vi "PH_Beckhoff_Application.declare digital PILS external InputTags.vi"() -> (0 "Digital Inputs":T2, 1 "Description":string)   [LabVIEW 2014, in "PH_Beckhoff_Application.lvlib"]
uses:
  PH_Beckhoff_Application.lvlib
  PH_Beckhoff/PH_Beckhoff.Digital Inputs.ctl
  PH_Beckhoff/PH_Beckhoff.lvlib
panel:
  in  "Digital Input Value":T1
  out "Right Size?":bool
  # "Let this VI run to check the size!"
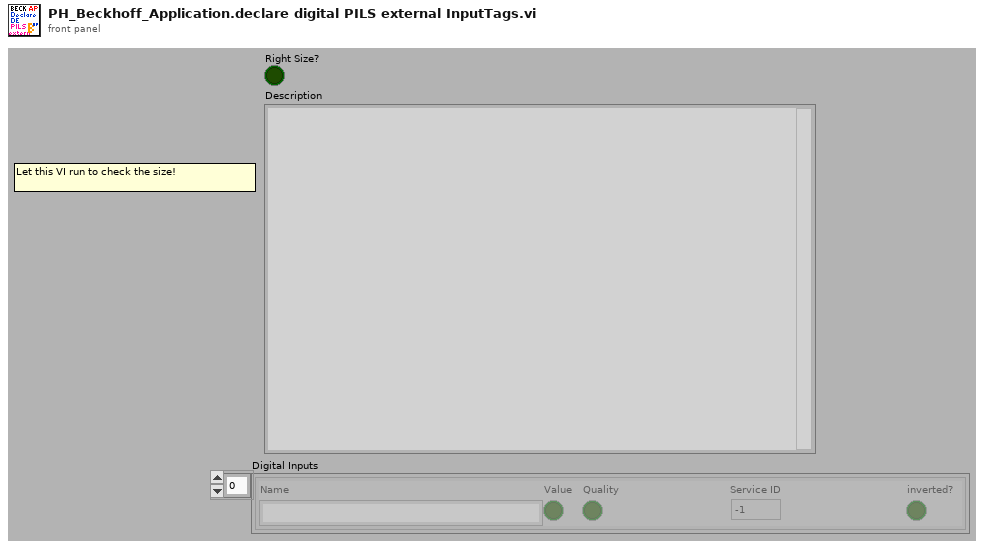
[diagram p1: front panel]
types:
  T1 = cluster{"Name":string, "Value":bool, "Quality":bool, "Service ID":i32, "inverted?":bool}
  T2 = typedef "PH_Beckhoff.lvlib/PH_Beckhoff.Digital Inputs.ctl" = cluster{"Name":string, "Value":bool, "Quality":bool, "Service ID":i32, "inverted?":bool}[]
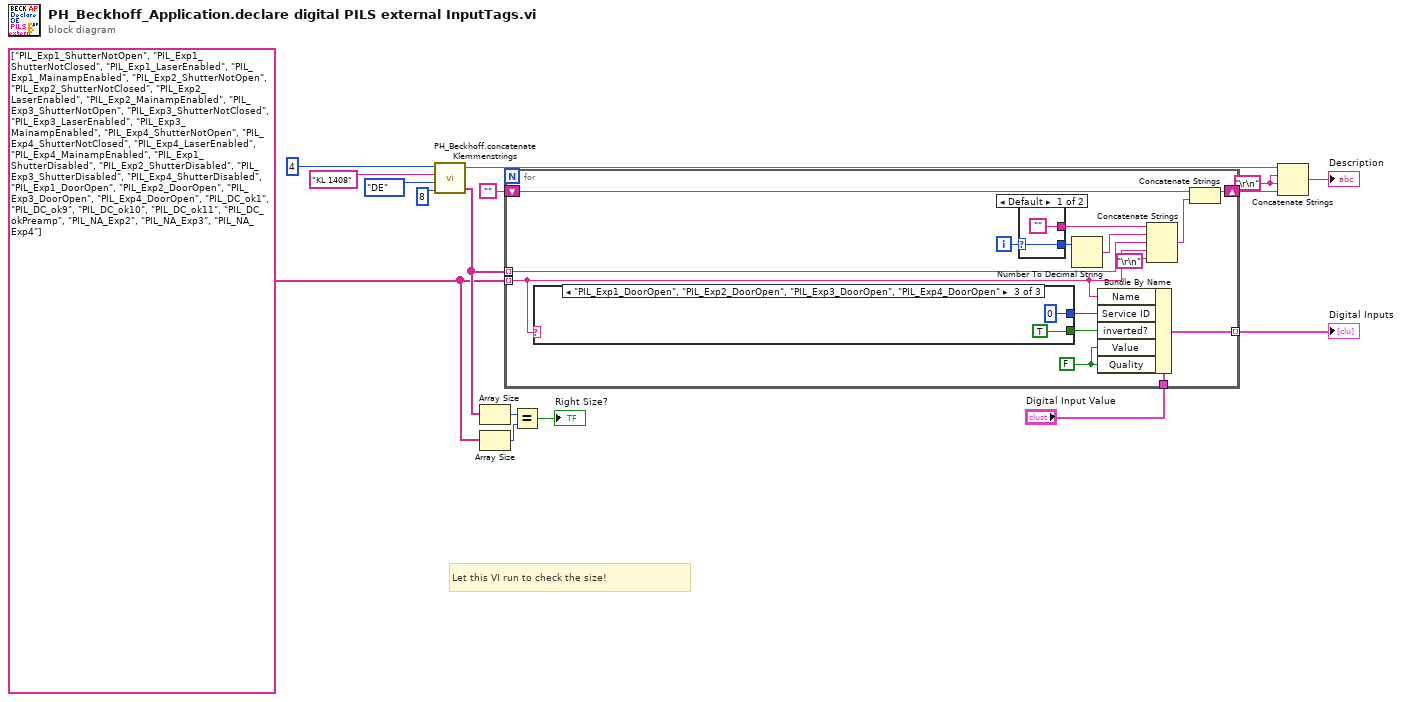
[diagram p0: block diagram]
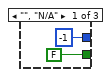
[diagram p2: hidden frame]
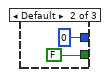
[diagram p3: hidden frame]
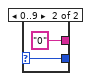
[diagram p4: hidden frame]
diagram:
  w2 = string[] ["PIL_Exp1_ShutterNotOpen", "PIL_Exp1_ShutterNotClosed", "PIL_Exp1_LaserEnabled", "PIL_Exp1_MainampEnabled", "PIL_Exp2_ShutterNotOpen", "PIL_Exp2_ShutterNotClosed", "PIL_Exp2_LaserEnabled", "PIL_Exp2_MainampEnabled", "PIL_Exp3_ShutterNotOpen", "PIL_Exp3_ShutterNotClosed", "PIL_Exp3_LaserEnabled", "PIL_Exp3_MainampEnabled", "PIL_Exp4_ShutterNotOpen", "PIL_Exp4_ShutterNotClosed", "PIL_Exp4_LaserEnabled", "PIL_Exp4_MainampEnabled", "PIL_Exp1_ShutterDisabled", "PIL_Exp2_ShutterDisabled", "PIL_Exp3_ShutterDisabled", "PIL_Exp4_ShutterDisabled", "PIL_Exp1_DoorOpen", "PIL_Exp2_DoorOpen", "PIL_Exp3_DoorOpen", "PIL_Exp4_DoorOpen", "PIL_DC_ok1", "PIL_DC_ok9", "PIL_DC_ok10", "PIL_DC_ok11", "PIL_DC_okPreamp", "PIL_NA_Exp2", "PIL_NA_Exp3", "PIL_NA_Exp4"] ("Array")
  w12 = "\r\n"
  # "Let this VI run to check the size!"
  n1 = call "PH_Beckhoff.concatenate Klemmenstrings.vi"("# of In- or Outputs"=8, "Type"=enum16{"AE", "AA", "DE", "DA"}."DE", "Klemmenname"="KL 1408", "Quantity"=4 ("size(s)")) -> ("concatenated string array"=w7:string[], "\"<Type>: <Quantity> x <Klemmenname>\""=w9:string)  [unwired: 1 out]
  n2 = Array Size(array=w7) -> (size(s)=w6:i32)
  n3 = Array Size(array=w2) -> (size(s)=w1:i32)
  n4 = for {
    tunnel: w2 -> [w17] mode=indexing
    tunnel: w7 -> [w27] mode=indexing
    shift-right: [w25] -> w13
    shift-left: "" -> [w24]
    tunnel: "Digital Input Value" -> [w23]
    tunnel: [w21] -> w3 mode=indexing
    i -> [w31]
    w20 = FALSE ("Quality")
    n5 = case shown="\"PIL_Exp1_DoorOpen\", \"PIL_Exp2_DoorOpen\", \"PIL_Exp3_DoorOpen\", \"PIL_Exp4_DoorOpen\"" w17 {
      tunnel: [-1 0 0] -> w22
      tunnel: [FALSE FALSE TRUE] -> w18
      frame "", "N/A" {
      }
      frame Default {
      }
      frame "PIL_Exp1_DoorOpen", "PIL_Exp2_DoorOpen", "PIL_Exp3_DoorOpen", "PIL_Exp4_DoorOpen" {
      }
    }
    n6 = case shown="Default" w31 {
      selector: w31 -> [w38 w41]
      tunnel: [w38 w41] -> w30
      tunnel: ["" "0"] -> w29
      frame Default {
      }
      frame 0..9 {
      }
    }
    n7 = Number To Decimal String(number=w30) -> (decimal integer string=w28:string)  [unwired: 1 in]
    n8 = Bundle By Name(cluster=w23, "Name"=w17, "Service ID"=w22, "inverted?"=w18, "Value"=w20, "Quality"=w20) -> (w21:T1)
    n9 = Concatenate Strings(w29, w28, w27, w17, "\r\n") -> (w26:string)
    n10 = Concatenate Strings(w24, w26) -> (w25:string)
  }
  "Digital Inputs" <- w3
  n11 = Equal?(x=w6, y=w1) -> (x = y?=→"Right Size?":bool)
  n12 = Concatenate Strings(w9, w12, w12, w13) -> (→"Description":string)
